vi "Close Module.vi"(8 "error in":errorcluster, 9 "Wait for stop?":bool, 11 "Module Admin in":refnum<class "Delacor_lib_QMH_Cloneable Module Admin.lvclass">) -> (0 "error out":errorcluster, 1 "External Launch":bool, 3 "Module Admin out":refnum<class "Delacor_lib_QMH_Cloneable Module Admin.lvclass">)   [LabVIEW 2018, in "ModuleInterface.lvlib"]
doc: "Destroy the Broadcast Events and Request Events (if this was the first instance). Reset flags stored in Module Admin class.\n_____\nBased on DQMH Project Template 7.0.1.1316."
uses:
  ModuleInterface.lvlib
  <vilib>/Delacor/Delacor QMH/Libraries/Cloneable Module Admin_class/Delacor_lib_QMH_Cloneable Module Admin.lvclass
  C:/Program Files (x86)/National Instruments/LabVIEW 2018/vi.lib/Delacor/Delacor QMH/Libraries/Module Admin_class/Delacor_lib_QMH_Module Admin.lvclass
  Stop Argument--cluster.ctl
  <vilib>/Delacor/Delacor QMH/Libraries/Cloneable Module Admin_class/Delacor_lib_QMH_Cloneable Module Admin.lvclass/Delacor_lib_QMH_Cloneable Module Admin.ctl
  <vilib>/Delacor/Delacor QMH/Libraries/Module Admin_class/Delacor_lib_QMH_Module Admin.lvclass/Delacor_lib_QMH_Module Admin.ctl
  <vilib>/Delacor/Delacor QMH/Libraries/Cloneable Module Admin_class/Delacor_lib_QMH_Get First.vi
  <vilib>/Delacor/Delacor QMH/Libraries/Cloneable Module Admin_class/Delacor_lib_QMH_Get Module ID.vi
  <vilib>/Delacor/Delacor QMH/Libraries/Module Admin_class/Delacor_lib_QMH_Get External Launch.vi
  <vilib>/Delacor/Delacor QMH/Libraries/Cloneable Module Admin_class/Delacor_lib_QMH_Get Close Master Reference.vi
  Clone Registration/Clone Registration.lvlib
  VI Reference Management/VI Reference Management.lvlib
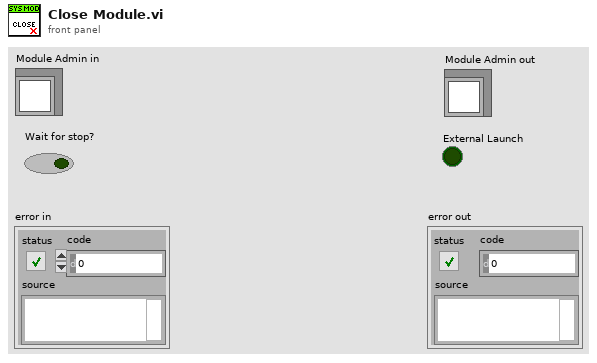
[diagram p1: front panel]
types:
  T1 = typedef "ModuleInterface.lvlib/Stop Argument--cluster.ctl" = cluster{"Module ID":i32, "Origin":string, "Exit via Stop Module Req?":bool, "Wait for Module to stop?":bool}
  T2 = typedef "Semaphore RefNum" = refnum<k1>
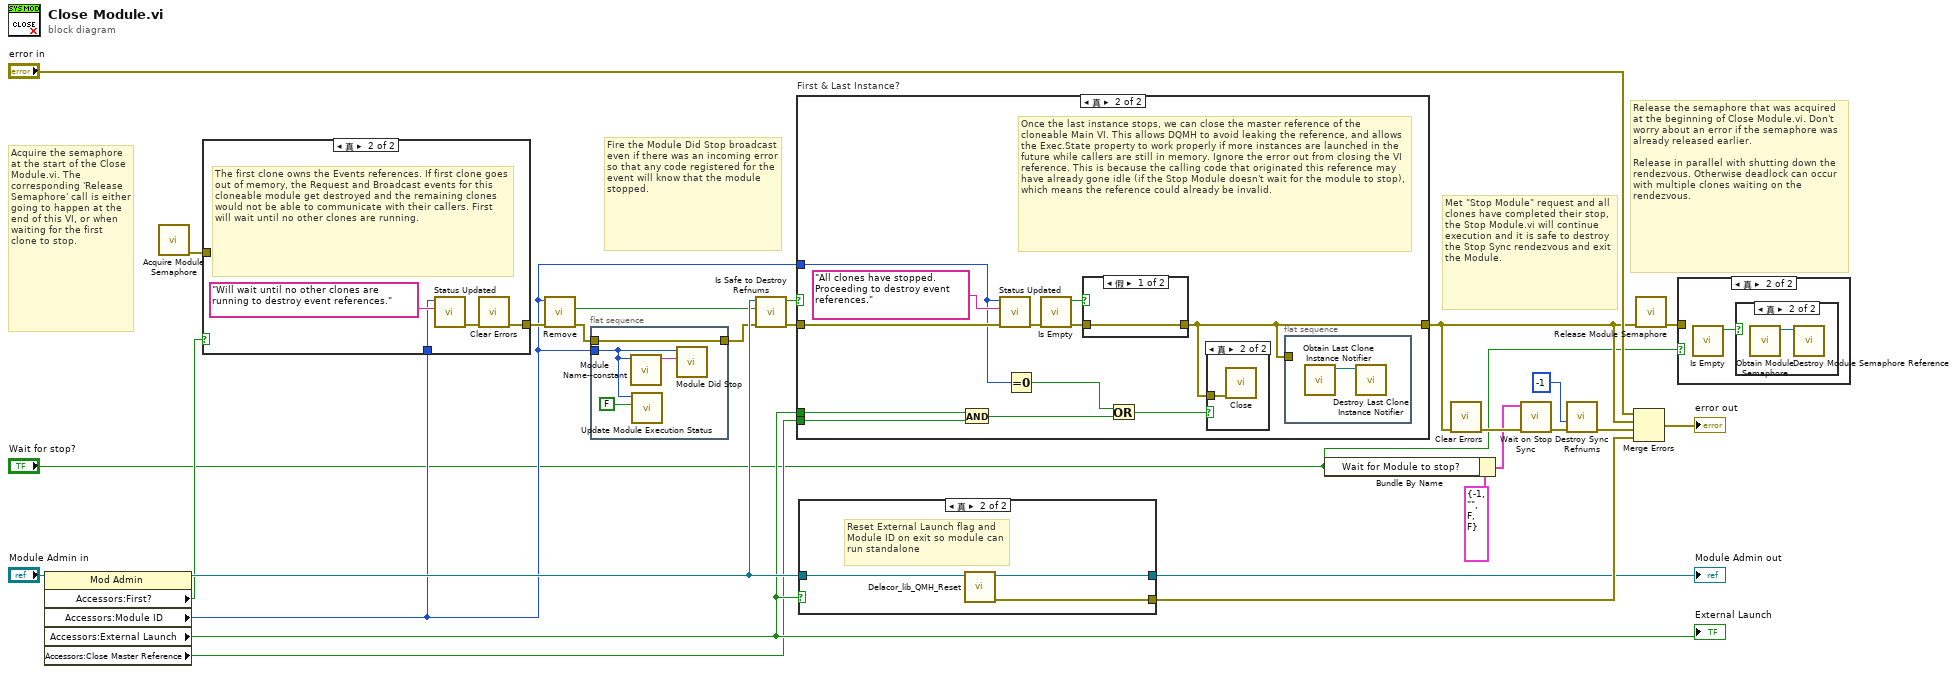
[diagram p0: block diagram]
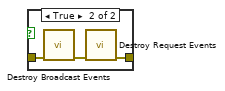
[diagram p7: hidden frame]
diagram:
  # "Release the semaphore that was acquired at the beginning of Close Module.vi. Don't worry about an error if the semaphore was already released earlier.\n\nRelease in parallel with shutting down the rendezvous. Otherwise deadlock can occur with multiple clones waiting on the rendezvous."
  # "Acquire the semaphore at the start of the Close Module.vi. The corresponding 'Release Semaphore' call is either going to happen at the end of this VI, or when waiting for the first clone to stop."
  # "Fire the Module Did Stop broadcast even if there was an incoming error so that any code registered for the event will know that the module stopped."
  # "Met \"Stop Module\" request and all clones have completed their stop, the Stop Module.vi will continue execution and it is safe to destroy the Stop Sync rendezvous and exit the Module."
  n1 = property class="Mod Admin"(reference="Module Admin in") -> (reference out=w24:refnum<class "Delacor_lib_QMH_Cloneable Module Admin.lvclass">, "Accessors:First?"=w15:bool, "Accessors:Module ID"=w9:i32, "Accessors:External Launch"=w13:bool, "Accessors:Close Master Reference"=w8:bool)  [unwired: 1 in, 1 out]
  "External Launch" <- w13
  n2 = call "Acquire Module Semaphore.vi"() -> ("error out"=w7:errorcluster)  [unwired: 11 in]
  n3 = case shown="真" w15 {
    tunnel: w9 -> [_ w29]
    tunnel: [_ w27] -> w26
    tunnel: w7 -> [_ _]
    frame False {
    }
    frame True {
      # "The first clone owns the Events references. If first clone goes out of memory, the Request and Broadcast events for this cloneable module get destroyed and the remaining clones would not be able to communicate with their callers. First will wait until no other clones are running."
      n4 = call "Status Updated.vi"("Status"="Will wait until no other clones are running to destroy event references." ("format string"), "Module ID"=w29) -> ("error out"=w28:errorcluster)  [unwired: 9 in]
      n5 = call <vilib>:"Clear Errors.vi"("error in (no error)"=w28) -> ("error out"=w27:errorcluster)  [unwired: 5 in, 1 out]
    }
  }
  n6 = call "Remove.vi"("error in"=w26, "Module ID"=w9) -> ("error out"=w11:errorcluster, "empty"=w12:bool)  [unwired: 8 in]
  n7 = flat-sequence {
    tunnel: w11 -> [w34]
    tunnel: [w34] -> w10
    tunnel: w9 -> [w32]
    frame #0 {
      n8 = call "Module Name--constant.vi"("Module ID"=w32) -> ("Module Name"=w33:string)  [unwired: 10 in]
      n9 = call "Update Module Execution Status.vi"("Running?"=FALSE, "Module ID"=w32) -> ()  [unwired: 9 in, 1 out]
      n10 = call "Module Did Stop.vi"("Origin"=w33, "Module ID"=w32) -> ()  [unwired: 9 in, 1 out]
    }
  }
  n11 = call "Is Safe to Destroy Refnums.vi"("error in"=w10, "empty"=w12, "Module Admin"=w24) -> ("error out"=w21:errorcluster, "Destroy Broadcast & Request Event Refs?"=w22:bool)  [unwired: 7 in]
  n12 = case "First & Last Instance?" shown="真" w22 {
    tunnel: w21 -> [w35 w47]
    tunnel: [w35 w39] -> w5
    tunnel: w9 -> [_ w41]
    tunnel: w13 -> [_ w45]
    tunnel: w8 -> [_ w43]
    frame False {
    }
    frame True {
      # "Once the last instance stops, we can close the master reference of the cloneable Main VI. This allows DQMH to avoid leaking the reference, and allows the Exec.State property to work properly if more instances are launched in the future while callers are still in memory. Ignore the error out from closing the VI reference. This is because the calling code that originated this reference may have already gone idle (if the Stop Module doesn't wait for the module to stop), which means the reference could already be invalid."
      n13 = And(x=w45, y=w43) -> (x .and. y?=w44:bool)
      n14 = call "Status Updated.vi"("error in"=w47, "Status"="All clones have stopped. Proceeding to destroy event references.", "Module ID"=w41) -> ("error out"=w38:errorcluster)  [unwired: 8 in]
      n15 = Equal To 0?(x=w41) -> (x = 0?=w40:bool)
      n16 = call "Is Empty.vi"("error in"=w38) -> ("error out"=w37:errorcluster, "Empty?"=w36:bool)  [unwired: 9 in]
      n17 = case shown="假" w36 {
        tunnel: [w48 w50] -> w39
        tunnel: w37 -> [w48 w49]
        frame False {
        }
        frame True {
          n18 = call "Destroy Broadcast Events.vi"("error in"=w49) -> ("error out"=w51:errorcluster)  [unwired: 10 in]
          n19 = call "Destroy Request Events.vi"("error in"=w51) -> ("error out"=w50:errorcluster)  [unwired: 10 in]
        }
      }
      n20 = Or(x=w40, y=w44) -> (x .or. y?=w42:bool)
      n21 = case shown="真" w42 {
        tunnel: w39 -> [_ w53]
        frame False {
        }
        frame True {
          n22 = call "Close.vi"("error in"=w53) -> ()  [unwired: 10 in, 1 out]
        }
      }
      n23 = flat-sequence {
        tunnel: w39 -> [_]
        frame #0 {
          n24 = call "Obtain Last Clone Instance Notifier.vi"() -> ("Last Instance Notifier"=w52:refnum<notifier>)  [unwired: 10 in, 1 out]
          n25 = call "Destroy Last Clone Instance Notifier.vi"("Last Instance Notifier"=w52) -> ()  [unwired: 11 in]
        }
      }
    }
  }
  n26 = case shown="真" w13 {
    tunnel: w24 -> [w54 w57]
    tunnel: [w54 w56] -> w20
    tunnel: [_ w55] -> w25
    frame False {
    }
    frame True {
      # "Reset External Launch flag and Module ID on exit so module can run standalone"
      n27 = call-dynamic "Delacor_lib_QMH_Reset.vi"("Mod Admin in"=w57) -> ("error out"=w55:errorcluster, "Mod Admin out"=w56:refnum<class "Delacor_lib_QMH_Cloneable Module Admin.lvclass">)  [unwired: 9 in]
    }
  }
  "Module Admin out" <- w20
  n28 = Bundle By Name(cluster=T1 {"Module ID"=-1, "Origin"="", "Exit via Stop Module Req?"=FALSE, "Wait for Module to stop?"=FALSE} ("Stop Argument"), "Wait for Module to stop?"="Wait for stop?") -> (w2:T1)
  n29 = call <vilib>:"Clear Errors.vi"("error in (no error)"=w5) -> ("error out"=w16:errorcluster)  [unwired: 5 in, 1 out]
  n30 = call "Wait on Stop Sync.vi"("error in"=w16, "Stop Argument"=w2) -> ("error out"=w19:errorcluster)  [unwired: 9 in]
  n31 = call "Destroy Sync Refnums.vi"("error in"=w19, "Module ID"=-1) -> ("error out"=w18:errorcluster)  [unwired: 9 in]
  n32 = Merge Errors("error in", w5, w18, w25) -> (→"error out":errorcluster)
  n33 = call "Release Module Semaphore.vi"("error in"=w5) -> ("error out"=w4:errorcluster)  [unwired: 10 in]
  n34 = case shown="真" "Wait for stop?" {
    tunnel: w4 -> [_ _]
    frame False {
    }
    frame True {
      n35 = call "Is Empty.vi"() -> ("Empty?"=w58:bool)  [unwired: 10 in, 1 out]
      n36 = case shown="真" w58 {
        frame False {
        }
        frame True {
          n37 = call "Obtain Module Semaphore.vi"() -> ("semaphore"=w59:T2)  [unwired: 9 in, 2 out]
          n38 = call "Destroy Module Semaphore Reference.vi"("semaphore"=w59) -> ()  [unwired: 10 in, 1 out]
        }
      }
    }
  }
